vi "ep_Calculate Symmetrical Components.vi"(0 "line voltage? (F)":bool, 2 "cycles per block":i32, 5 "error in (no error)":errorcluster, 6 "voltage complex spectra (5Hz step)":T2(array[cluster]), 7 "current complex spectra (5Hz step)":T2(array[cluster])) -> (10 "voltage":dbl[](array[numeric]), 12 "fundamental voltage":dbl[](array[numeric]), 14 "current":dbl[](array[numeric]), 15 "fundamental current":dbl[](array[numeric]), 16 "active power":dbl[](array[numeric]), 17 "fundamental active power":dbl[](array[numeric]), 18 "fundamental reactive power":dbl[](array[numeric]), 19 "error out":errorcluster)   [LabVIEW 2014, in "NI_EP_Power Quality.lvlib"]
uses:
  <vilib>/addons/Electrical Power/PQ/NI_EP_Power Quality.lvlib
  <vilib>/addons/Electrical Power/PQ/Common/Controls/ep_AI Data Channel.ctl
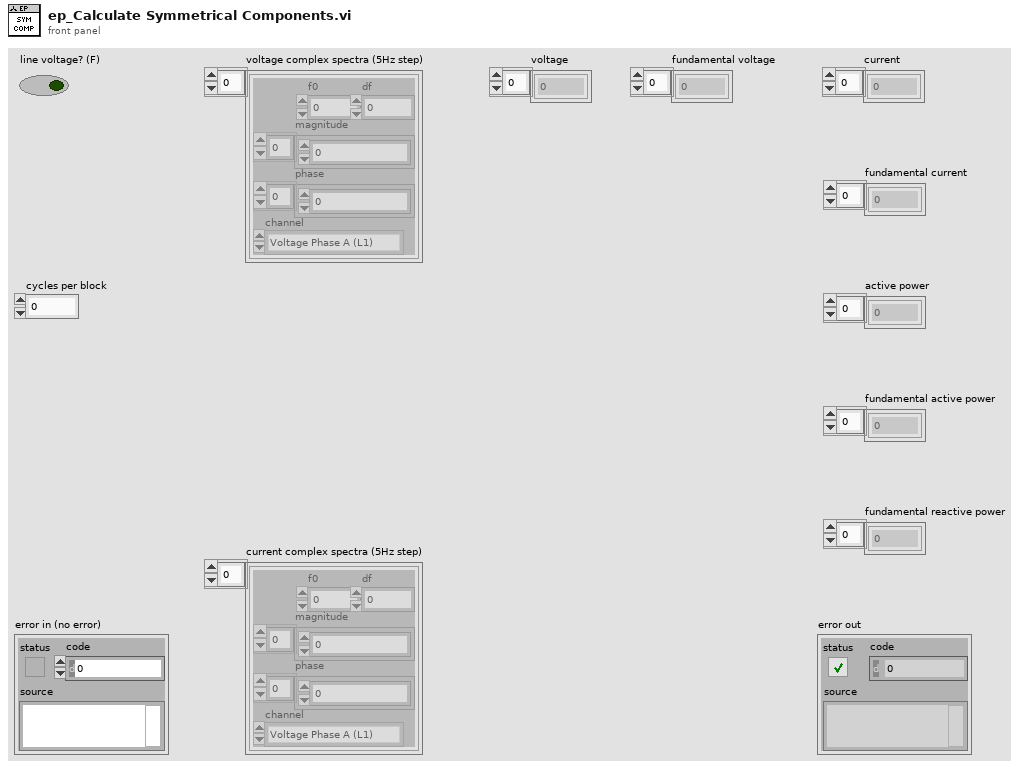
[diagram p1: front panel]
types:
  T1 = typedef "NI_EP_Power Quality.lvlib/ep_AI Data Channel.ctl" = enum16{"Voltage Phase A (L1)", "Voltage Phase B (L2)", "Voltage Phase C (L3)", "Voltage Phase N (Neutral)", "Current Phase A (L1)", "Current Phase B (L2)", "Current Phase C (L3)", "Current Phase N (Neutral)"}
  T2 = cluster{"f0":dbl, "df":dbl, "magnitude":dbl[], "phase":dbl[], "channel":T1}[]
  T3 = cluster{"zero":cdb[], "positive":cdb[], "negative":cdb[]}
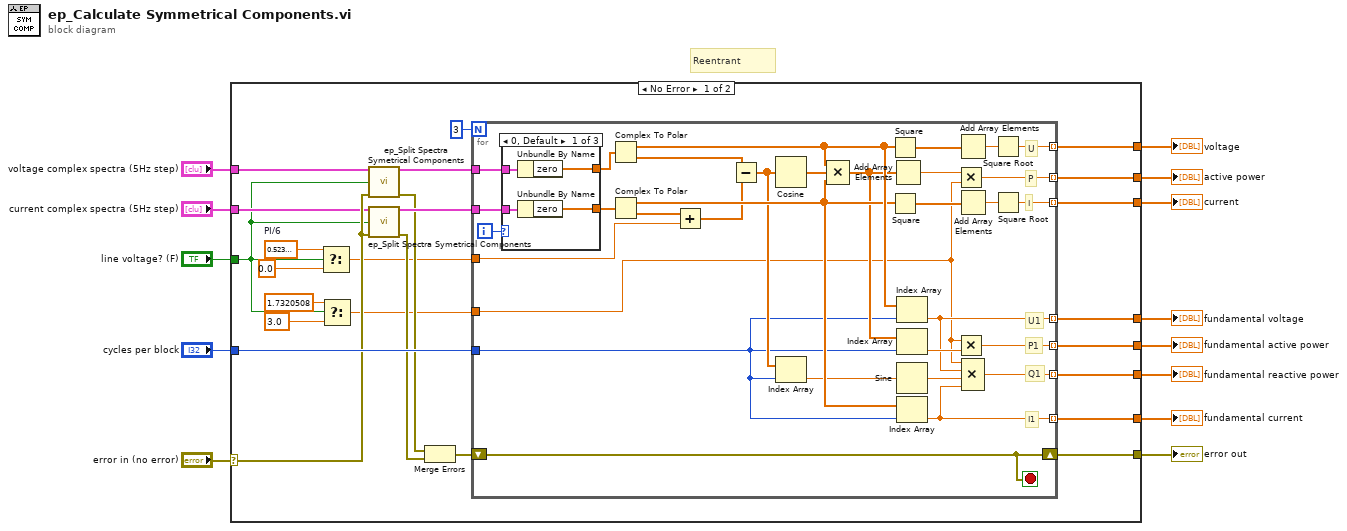
[diagram p0: block diagram]
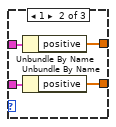
[diagram p2: hidden frame]
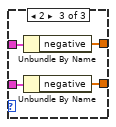
[diagram p3: hidden frame]
diagram:
  # "Reentrant"
  n1 = case shown="No Error" "error in (no error)" {
    selector: "error in (no error)" -> [w34 w83]
    tunnel: "cycles per block" -> [w35 _]
    tunnel: [w30 w83] -> w11
    tunnel: "voltage complex spectra (5Hz step)" -> [w29 _]
    tunnel: "current complex spectra (5Hz step)" -> [w28 _]
    tunnel: [w27 _] -> w8
    tunnel: [w26 _] -> w7
    tunnel: [w25 _] -> w6
    tunnel: [w24 _] -> w5
    tunnel: [w23 _] -> w4
    tunnel: [w22 _] -> w3
    tunnel: [w21 _] -> w2
    tunnel: "line voltage? (F)" -> [w15 _]
    frame No Error {
      w19 = 0.5235987755982988  # PI/6
      n2 = Select(t=w19, s=w15, f=0.0) -> (s? t:f=w17:dbl)
      n3 = Select(t=1.7320508 ("x"), s=w15, f=3.0 ("x")) -> (s? t:f=w16:dbl)
      n4 = call <vilib>:"ep_Split Spectra Symetrical Components.vi"("complex spectra (5Hz step)"=w29, "line voltage? (F)"=w15, "error in (no error)"=w34) -> ("spectra symetrical components"=w37:T3, "error out"=w33:errorcluster)  [unwired: 11 in]
      n5 = call <vilib>:"ep_Split Spectra Symetrical Components.vi"("complex spectra (5Hz step)"=w28, "line voltage? (F)"=w15, "error in (no error)"=w34) -> ("spectra symetrical components"=w36:T3, "error out"=w32:errorcluster)  [unwired: 11 in]
      n6 = Merge Errors(w33, w32) -> (w31:errorcluster)
      n7 = for {
        N: 3 -> [_]
        tunnel: w35 -> [w44]
        tunnel: [w56] -> w27 mode=indexing
        tunnel: [w55] -> w23 mode=indexing
        tunnel: [w54] -> w25 mode=indexing
        tunnel: [w53] -> w26 mode=indexing
        tunnel: [w52] -> w22 mode=indexing
        tunnel: [w51] -> w24 mode=indexing
        tunnel: [w50] -> w21 mode=indexing
        tunnel: w37 -> [w49]
        tunnel: w36 -> [w48]
        shift-right: [w41] -> w30
        shift-left: w31 -> [w41]
        tunnel: w16 -> [w40]
        tunnel: w17 -> [w39]
        i -> [w45]
        stop <- w41 stop-if-true
        # "Q1"
        # "P1"
        # "P"
        # "I1"
        # "I"
        # "U1"
        # "U"
        n8 = case shown="0, Default" w45 {
          tunnel: w49 -> [w74 w78 w82]
          tunnel: [w73 w77 w81] -> w47
          tunnel: w48 -> [w72 w76 w80]
          tunnel: [w71 w75 w79] -> w46
          frame 0, Default {
            n9 = Unbundle By Name(w74) -> ("zero"=w73:cdb[])
            n10 = Unbundle By Name(w72) -> ("zero"=w71:cdb[])
          }
          frame 1 {
            n11 = Unbundle By Name(w78) -> ("positive"=w77:cdb[])
            n12 = Unbundle By Name(w76) -> ("positive"=w75:cdb[])
          }
          frame 2 {
            n13 = Unbundle By Name(w82) -> ("negative"=w81:cdb[])
            n14 = Unbundle By Name(w80) -> ("negative"=w79:cdb[])
          }
        }
        n15 = Complex To Polar(r * e^(i*theta)=w47) -> (r=w63:dbl[], theta=w70:dbl[])
        n16 = Complex To Polar(r * e^(i*theta)=w46) -> (r=w62:dbl[], theta=w43:dbl[])
        n17 = Add(x=w43, y=w39) -> (x+y=w42:dbl[])
        n18 = Subtract(x=w70, y=w42) -> (x-y=w61:dbl[])
        n19 = Cosine(x=w61) -> (cos(x)=w64:dbl[])
        n20 = Index Array(array=w61, index=w44) -> (element=w60:dbl)
        n21 = Compound Arithmetic op=MULTIPLY(w63, w64, w62) -> (w59:dbl[])
        n22 = Square(x=w63) -> (x^2=w68:dbl[])
        n23 = Square(x=w62) -> (x^2=w66:dbl[])
        n24 = Add Array Elements(numeric array=w59) -> (sum=w65:dbl)
        n25 = Index Array(array=w63, index=w44) -> (element=w53:dbl)
        n26 = Index Array(array=w59, index=w44) -> (element=w58:dbl)
        n27 = Sine(x=w60) -> (sin(x)=w57:dbl)
        n28 = Index Array(array=w62, index=w44) -> (element=w51:dbl)
        n29 = Multiply(x=w65, y=w40) -> (x*y=w55:dbl)
        n30 = Multiply(x=w40, y=w58) -> (x*y=w52:dbl)
        n31 = Add Array Elements(numeric array=w68) -> (sum=w69:dbl)
        n32 = Add Array Elements(numeric array=w66) -> (sum=w67:dbl)
        n33 = Compound Arithmetic op=MULTIPLY(w40, w53, w57, w51) -> (w50:dbl)
        n34 = Square Root(x=w69) -> (sqrt(x)=w56:dbl)
        n35 = Square Root(x=w67) -> (sqrt(x)=w54:dbl)
      }
    }
    frame Error {
    }
  }
  "error out" <- w11
  "voltage" <- w8
  "fundamental voltage" <- w7
  "current" <- w6
  "fundamental current" <- w5
  "active power" <- w4
  "fundamental active power" <- w3
  "fundamental reactive power" <- w2
